vi "freq_counter_standalone.vi"() -> ()   [LabVIEW 2013]
panel:
  out "SetRange":i16
  in  "Get Frequency":bool
  in  "stop":bool
  out "Frequency":dbl
  in  "Range":dbl
  in  "Sampling Time":dbl
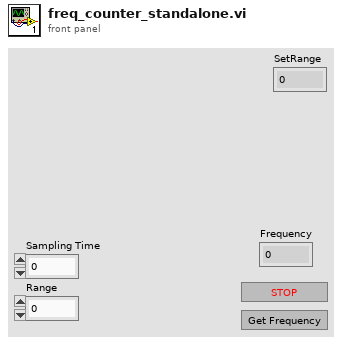
[diagram p1: front panel]
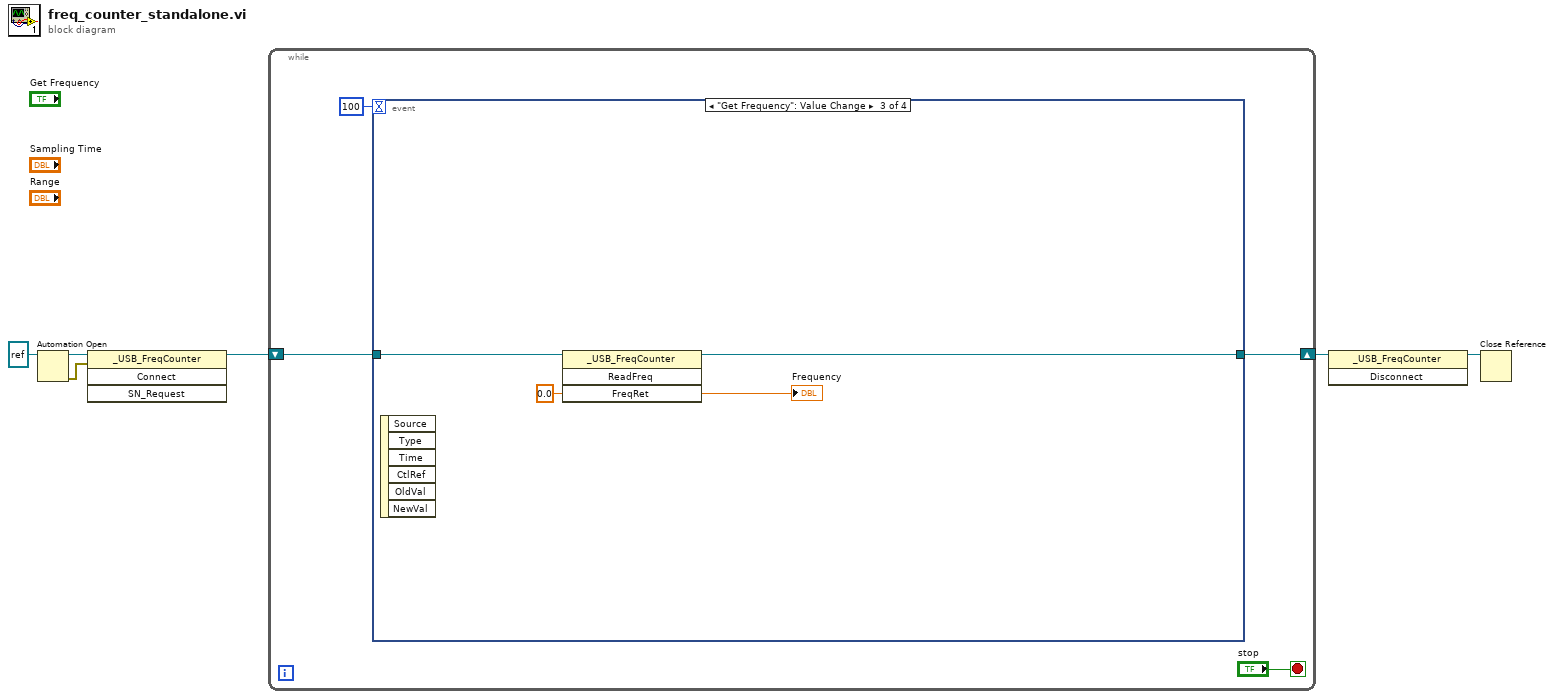
[diagram p0: block diagram]
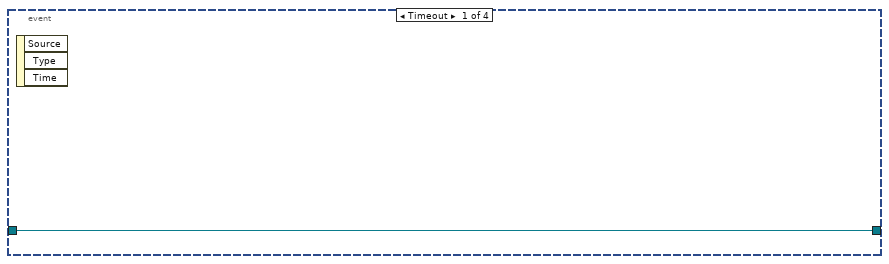
[diagram p2: hidden frame]
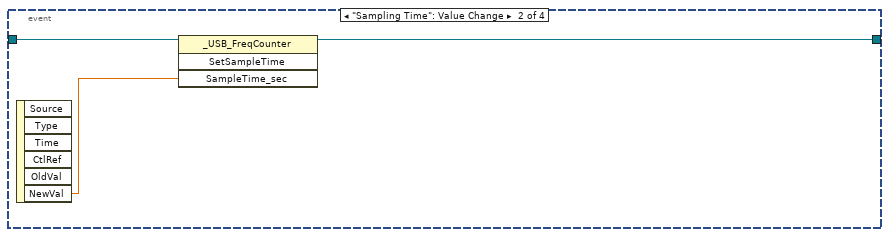
[diagram p3: hidden frame]
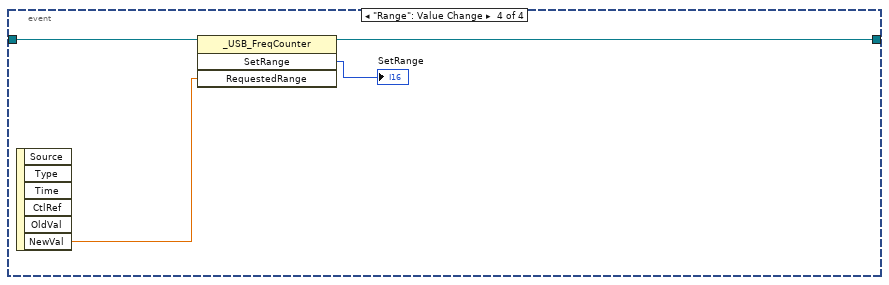
[diagram p4: hidden frame]
diagram:
  n1 = Automation Open(Automation Refnum=refnum<k7> refnum ("MCL_FreqCounter._USB_FreqCounter")) -> (Automation Refnum=w5:refnum<k7>, error out=w4:errorcluster)  [unwired: 3 in]
  n2 = invoke class="_USB_FreqCounter" method="Connect"(reference=w5, error in=w4) -> (reference out=w3:refnum<k7>)  [unwired: 2 in, 3 out]
  n3 = while {
    shift-right: [w7] -> w2
    shift-left: w3 -> [w8]
    stop <- "stop" stop-if-true
    n4 = event shown="[2] \"Get Frequency\": Value Change" {
      selector: _ -> [_ _ _ _]
      dyn-events: _ -> [_ _ _ _]
      timeout: 100 -> [_ _ _ _]
      tunnel: w8 -> [w11 w14 w18 w21]
      tunnel: [w11 w12 w16 w19] -> w7
      event Timeout {
        n5 = event-data() -> ()  [unwired: 1 in, 3 out]
      }
      event "Sampling Time": Value Change {
        n6 = event-data() -> ("NewVal"=w13:dbl)  [unwired: 1 in, 5 out]
        n7 = invoke class="_USB_FreqCounter" method="SetSampleTime"(reference=w14, "SampleTime_sec"=w13) -> (reference out=w12:refnum<k7>)  [unwired: 2 in, 3 out]
      }
      event "Get Frequency": Value Change {
        n8 = event-data() -> ()  [unwired: 1 in, 6 out]
        n9 = invoke class="_USB_FreqCounter" method="ReadFreq"(reference=w18, "FreqRet"=0.0) -> (reference out=w16:refnum<k7>, "FreqRet"=→"Frequency":dbl)  [unwired: 2 in, 2 out]
      }
      event "Range": Value Change {
        n10 = event-data() -> ("NewVal"=w22:dbl)  [unwired: 1 in, 5 out]
        n11 = invoke class="_USB_FreqCounter" method="SetRange"(reference=w21, "RequestedRange"=w22) -> (reference out=w19:refnum<k7>, "SetRange"=→"SetRange":i16)  [unwired: 2 in, 2 out]
      }
    }
  }
  n12 = invoke class="_USB_FreqCounter" method="Disconnect"(reference=w2) -> (reference out=w1:refnum<k7>)  [unwired: 2 in, 2 out]
  n13 = Close Reference(reference=w1) -> ()  [unwired: 1 in, 1 out]
